vi "CC Observation to Script.vi"(8 "error in (no error)":errorcluster, 11 "Observation":T3={"Priority"=0, "ID"="", "Observer"="", "Obj Name"="", "Obj Type"="", "RA and DEC String"={"RA"="HH:MM:SS.nnn", "DEC"="DEG:arcmin:arcsec.nn"}, "Filters"=[], "Integration Time"=0.0, "Observation Status"=enum."Error", "Offsets"={"RA"=0.0, "DEC"=0.0, "ROT"=0.0}, "Images"=0, "Dither Options"={"Dither"=enum."None", "Dither Radius"=0.0, "Dither Points"=0, "Dither Phase"=0.0, "B Offset"={"RA"=0.0, "DEC"=0.0}}, "Comment 1"="", "Comment 2"=""}) -> (0 "error out":errorcluster, 3 "Script Steps":T1[](array[typedef]))   [LabVIEW 2024]
uses:
  typedefs/CC cluster Observation.ctl
  Observation Queue/CC enum Observation Status.ctl
  Telescope/CC cluster Telescope Offsets.ctl
  typedefs/CC cluster Observation Dither Options.ctl
  typedefs/CC enum Dither Selection.ctl
  typedefs/CC cluster RA and DEC.ctl
  typedefs/CC Script Step.ctl
  typedefs/CC enum Script Action.ctl
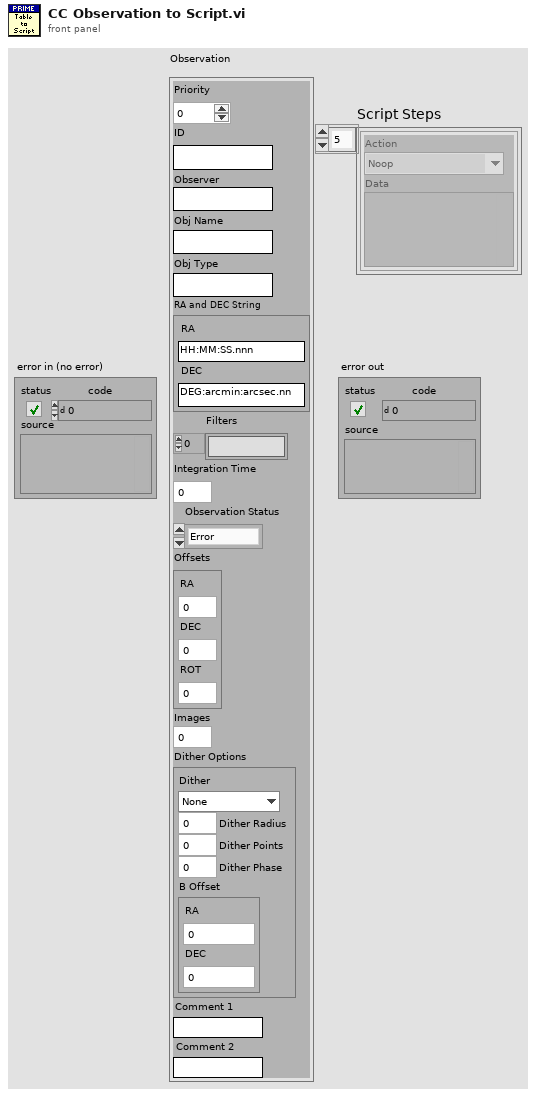
[diagram p1: front panel]
types:
  T1 = typedef "CC Script Step.ctl" = cluster{"Action":T2, "Data":variant}
  T2 = typedef "CC enum Script Action.ctl" = enum16{"Noop", "Define Object", "Define Exposure", "Define Dithering", "Acquire Images", "Set Filter Wheel", "Telescope Home", "Telescope Move", "Telescope RA DEC", "Focus Move Relative", "Focus Move Absolute", "Focus Set Home", "Macro", "Pause", "Ask User", "Define Random Dither", "CmdLine", "Outlet"}
  T3 = typedef "CC cluster Observation.ctl" = cluster{"Priority":i32, "ID":string, "Observer":string, "Obj Name":string, "Obj Type":string, "RA and DEC String":cluster{"RA":string, "DEC":string}, "Filters":string[], "Integration Time":dbl, "Observation Status":T4, "Offsets":T5, "Images":i32, "Dither Options":T6, "Comment 1":string, "Comment 2":string}
  T4 = typedef "CC enum Observation Status.ctl" = enum16{"Ready", "Running", "Done", "Error"}
  T5 = typedef "CC cluster Telescope Offsets.ctl" = cluster{"RA":dbl, "DEC":dbl, "ROT":dbl}
  T6 = typedef "CC cluster Observation Dither Options.ctl" = cluster{"Dither":T7, "Dither Radius":dbl, "Dither Points":i32, "Dither Phase":dbl, "B Offset":T8}
  T7 = typedef "CC enum Dither Selection.ctl" = enum16{"None", "Circle", "Random", "ABBA"}
  T8 = typedef "CC cluster RA and DEC.ctl" = cluster{"RA":dbl, "DEC":dbl}
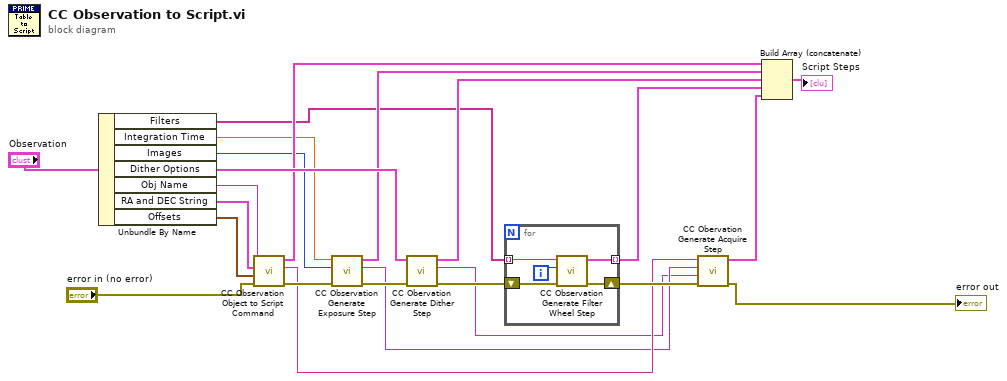
[diagram p0: block diagram]
diagram:
  n1 = Unbundle By Name("Observation") -> ("Filters"=w1:string[], "Integration Time"=w17:dbl, "Images"=w2:i32, "Dither Options"=w20:T6, "Obj Name"=w13:string, "RA and DEC String"=w14:cluster{"RA":string, "DEC":string}, "Offsets"=w15:T5)
  n2 = call "CC Observation Object to Script Command.vi"("error in (no error)"="error in (no error)", "Offsets"=w15, "RA and DEC String"=w14, "Object.Name"=w13) -> ("error out"=w12:errorcluster, "Object Name out"=w5:string, "Define Object Step"=w19:T1)  [unwired: 5 in]
  n3 = call "CC Observation Generate Exposure Step.vi"("error in (no error)"=w12, "Images"=w2, "Integration Time"=w17) -> ("error out"=w11:errorcluster, "Exp Name"=w4:string, "Exp Step"=w16:T1)  [unwired: 6 in]
  n4 = call "CC Obervation Generate Dither Step.vi"("error in (no error)"=w11, "Dither Options"=w20) -> ("error out"=w10:errorcluster, "Name"=w3:string, "Step"=w21:T1)  [unwired: 7 in]
  n5 = for {
    tunnel: w1 -> [w28] mode=indexing
    tunnel: [w26] -> w18 mode=indexing
    shift-right: [w24] -> w8
    shift-left: w10 -> [w25]
    i -> [w27]
    n6 = call "CC Observation Generate Filter Wheel Step.vi"("error in (no error)"=w25, "Wheel (0 or 1)"=w27, "Filter Wheel Name"=w28) -> ("error out"=w24:errorcluster, "Step"=w26:T1)  [unwired: 7 in]
  }
  n7 = call "CC Obervation Generate Acquire Step.vi"("error in (no error)"=w8, "Dithering"=w3, "Exposure"=w4, "Object"=w5) -> ("error out"=→"error out":errorcluster, "Acquire Step"=w6:T1)  [unwired: 6 in]
  n8 = Build Array (concatenate)(w19, w16, w21, w18, w6) -> (→"Script Steps":T1[])
